vi "Main.vi"() -> ()   [LabVIEW 2011]
panel:
  in  "stop":bool
  out "Delayed Output":bool
  in  "Interval (ms)":u32=1000
  in  "Input":bool
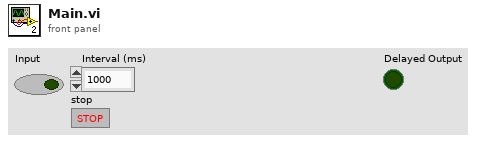
[diagram p1: front panel]
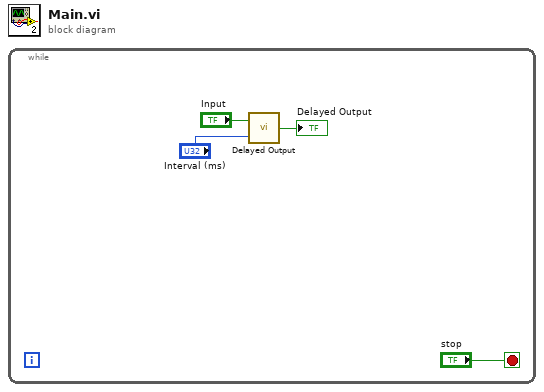
[diagram p0: block diagram]
diagram:
  n1 = while {
    stop <- "stop" stop-if-true
    n2 = call "Delayed Output.vi"("Interval (ms)"="Interval (ms)", "Input"="Input") -> ("Delayed Output"=→"Delayed Output":bool)
  }
